vi "13.模拟信号触发.vi"() -> ()   [LabVIEW 2019]
uses:
  <vilib>/rvi/Emulation/niFpgaGetClockAttributes.vi
  <vilib>/rvi/Emulation/niFpgaSctlEmulationGetInTimedLoop.vi
  <vilib>/rvi/Emulation/niFpgaEmulationReportErrorSimple.vi
  <vilib>/rvi/eio/common/nirviEmuTemplateMethod_errors.vi
  <vilib>/rvi/Emulation/niFpgaCriticalErrorInLSC.vi
  <vilib>/eio/EIONode/EIONode.xnode
  <vilib>/rvi/FXPMathLib/FxpInterpret/XNode/nifxpmath_Interpret.xnode
panel:
  out "x > y?":bool
  in  "Threshold":fxp<+/-,24,5>=2.0
  out "ConnectorA/AI1":fxp<+/-,24,5>
  in  "Count(Ticks)":u32=100 caption="计数器(滴答)"
  in  "采样点数":i32=1000 format="%.0p"
  in  "Trigger Level":fxp<+/-,24,5>=3.0
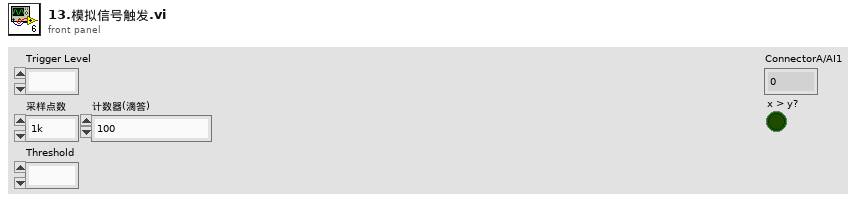
[diagram p1: front panel]
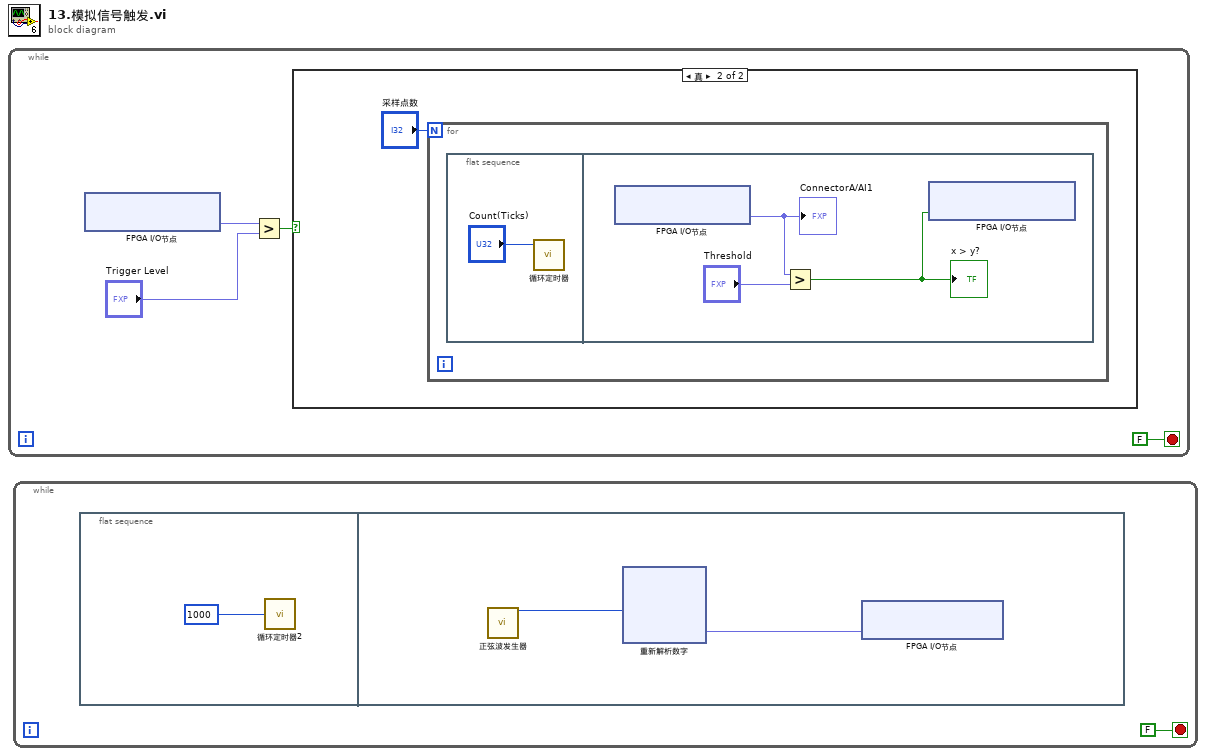
[diagram p0: block diagram]
diagram:
  n1 = while {
    stop <- FALSE stop-if-true
    n2 = xnode "FPGA I/O节点"() -> ("ConnectorB/AI0"=w4:fxp<+/-,24,5>)  [unwired: 1 in, 1 out]
    n3 = Greater?(x=w4, y="Trigger Level") -> (0:w2:bool)
    n4 = case shown="真" w2 {
      frame False {
      }
      frame True {
        n5 = for {
          N: "采样点数" -> [_]
          n6 = flat-sequence {
            frame #0 {
              n7 = call "循环定时器"("Count(Ticks)"="Count(Ticks)") -> ()  [unwired: 1 out]
            }
            frame #1 {
              n8 = xnode "FPGA I/O节点"() -> ("ConnectorA/AI1"=w9:fxp<+/-,24,5>)  [unwired: 1 in, 1 out]
              "ConnectorA/AI1" <- w9
              n9 = Greater?(x=w9, y="Threshold") -> (0:w7:bool)
              "x > y?" <- w7
              n10 = xnode "FPGA I/O节点"("ConnectorA/DIO8"=w7) -> ()  [unwired: 1 in, 1 out]
            }
          }
        }
      }
    }
  }
  n11 = while {
    stop <- FALSE stop-if-true
    n12 = flat-sequence {
      frame #0 {
        n13 = call "循环定时器2"("Count(Ticks)"=u32 1000) -> ()  [unwired: 1 out]
      }
      frame #1 {
        n14 = call "正弦波发生器"() -> ("sine out"=w13:i16)  [unwired: 15 in]
        n15 = xnode "重新解析数字"("x"=w13) -> ("y"=w12:fxp<+/-,16,4>)
        n16 = xnode "FPGA I/O节点"("ConnectorA/AO0"=w12) -> ()  [unwired: 1 in, 1 out]
      }
    }
  }
